vi "FCGI parse record header.vi"(11 "data":string) -> (3 "header":T1)   [LabVIEW 2013]
uses:
  FCGI record header.ctl
  FCGI record types.ctl
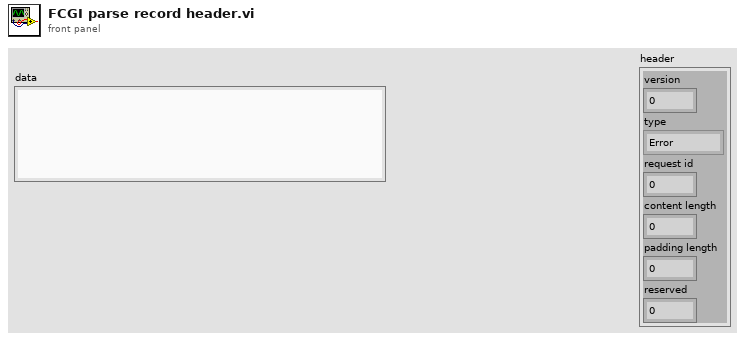
[diagram p1: front panel]
types:
  T1 = typedef "FCGI record header.ctl" = cluster{"version":u8, "type":T2, "request id":u16, "content length":u16, "padding length":u8, "reserved":u8}
  T2 = typedef "FCGI record types.ctl" = enum8{"Error", "Begin Request", "Abort Request", "End Request", "Parameters", "Standard Input", "Standard Output", "Standard Error", "Data", "Get Values", "Get Values Result", "Unknown Type"}
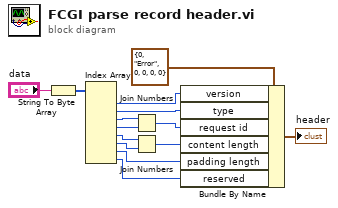
[diagram p0: block diagram]
diagram:
  n1 = String To Byte Array(string="data") -> (unsigned byte array=w13:u8[])
  n2 = Index Array(array=w13) -> (element #1=w11:u8, element #2=w10:u8, element #3=w9:u8, element #4=w8:u8, element #5=w6:u8, element #6=w5:u8, element #7=w3:u8, element #8=w2:u8)  [unwired: 8 in]
  n3 = Join Numbers(hi=w9, lo=w8) -> ((hi.lo)=w7:u16)
  n4 = Join Numbers(hi=w6, lo=w5) -> ((hi.lo)=w4:u16)
  n5 = Bundle By Name(cluster=T1 {"version"=0, "type"=enum."Error", "request id"=0, "content length"=0, "padding length"=0, "reserved"=0}, "version"=w11, "type"=w10, "request id"=w7, "content length"=w4, "padding length"=w3, "reserved"=w2) -> (→"header":T1)
